vi "PathCreate.vi"(7 "Location":enum16{"CUMC", "SERI", "VMR", "Aline", "HSS"}(ring)=enum."Aline", 9 "Probe Name":string, 10 "Patient Info":T1 {"Plane" min=1 max=12 step=1 scale=0.0..12.0}, 11 "base path":path) -> (1 "FileName":string, 3 "appended path":path)   [LabVIEW 2022 SP3]
uses:
  PatientInfoDef.ctl
panel:
  in  "Frequency":i16
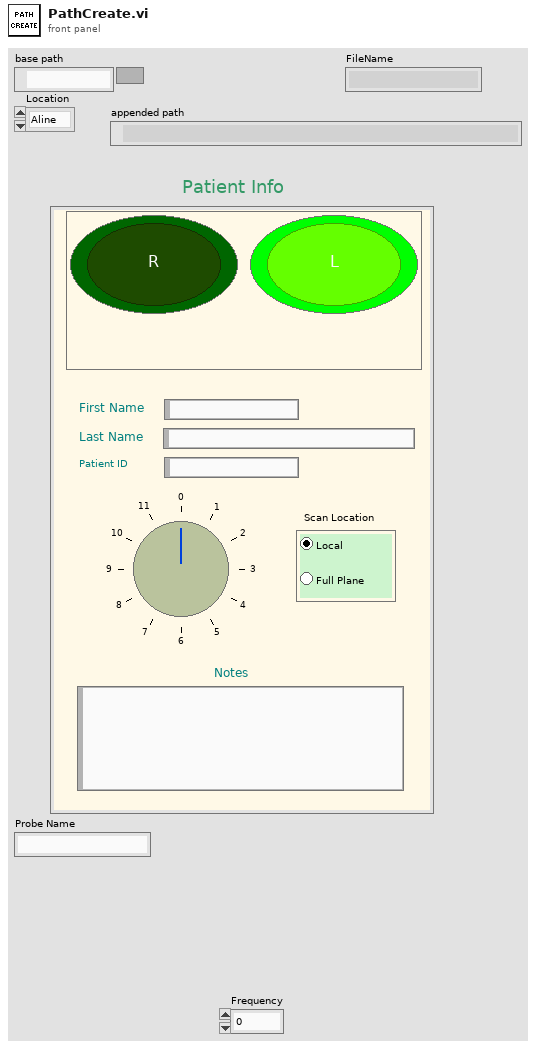
[diagram p1: front panel]
types:
  T1 = typedef "PatientInfoDef.ctl" = cluster{"Eye Selector":enum32{"Left", "Right"}, "Plane":i8, "First Name":string, "Last Name":string, "Notes":string, "Patient ID":string, "Scan Location":enum32{"Radio Selection 1", "Radio Selection 2"}}
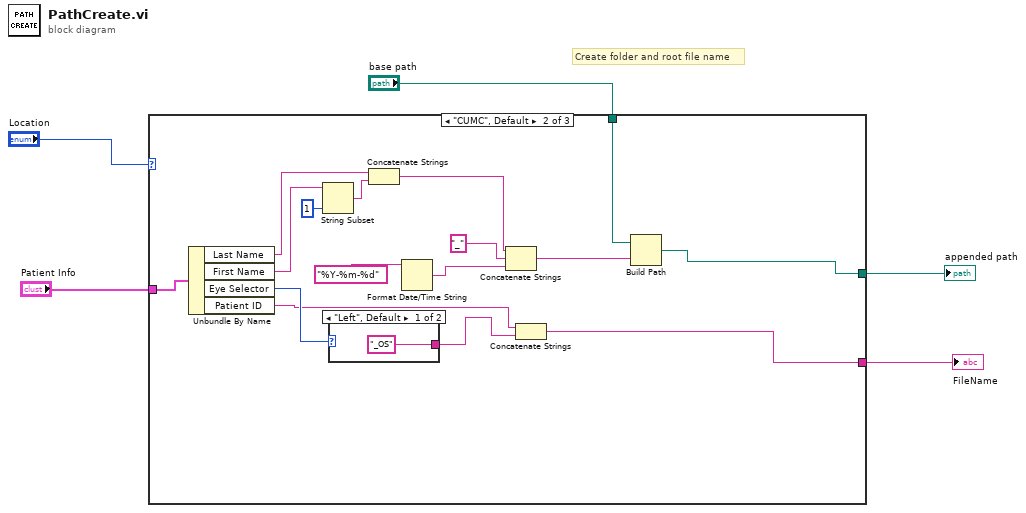
[diagram p0: block diagram]
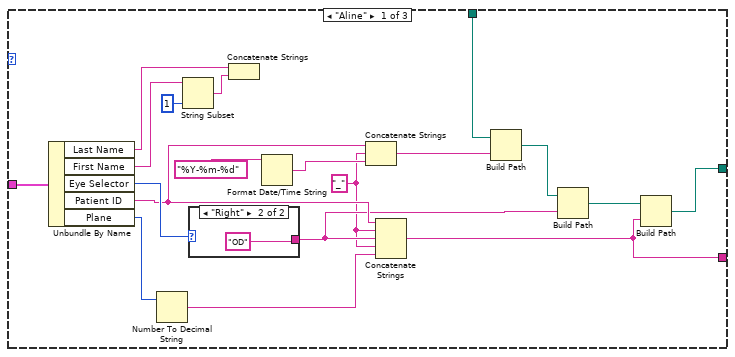
[diagram p2: hidden frame]
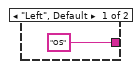
[diagram p3: hidden frame]
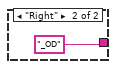
[diagram p4: hidden frame]
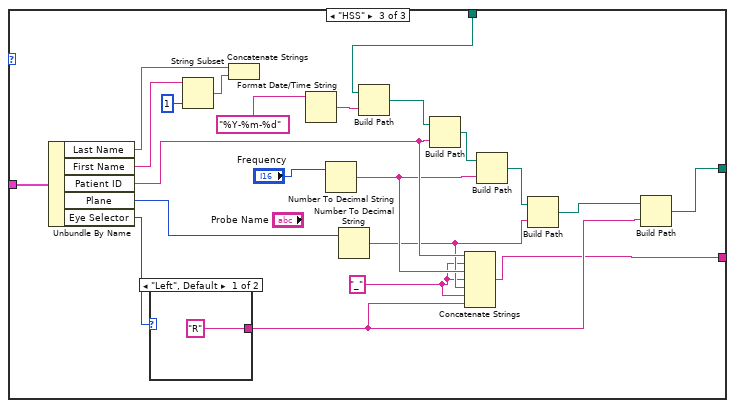
[diagram p5: hidden frame]
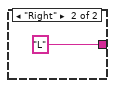
[diagram p6: hidden frame]
diagram:
  # "Create folder and root file name"
  n1 = case shown="\"CUMC\", Default" "Location" {
    tunnel: "base path" -> [w17 w35 w55]
    tunnel: "Patient Info" -> [w15 w33 w61]
    tunnel: [w7 w27 w58] -> w3
    tunnel: [w6 w30 w45] -> w2
    frame "Aline" {
      w9 = "_"
      n2 = Unbundle By Name(w15) -> ("Last Name"=w20:string, "First Name"=w22:string, "Eye Selector"=w23:enum32{"Left", "Right"}, "Patient ID"=w14:string, "Plane"=w11:i8)
      n3 = Number To Decimal String(number=w11) -> (decimal integer string=w10:string)  [unwired: 1 in]
      n4 = String Subset(string=w22, length (rest)=1 ("length (rest)")) -> (substring=w21:string)  [unwired: 1 in]
      n5 = case shown="\"Right\"" w23 {
        tunnel: ["OS" "OD"] -> w13
        frame "Left", Default {
        }
        frame "Right" {
        }
      }
      n6 = Concatenate Strings(w20, w21) -> ()  [unwired: 1 out]
      n7 = Format Date/Time String(time format string (%c)="%Y-%m-%d") -> (date/time string=w18:string)  [unwired: 2 in]
      n8 = Concatenate Strings(w14, w9, w18) -> (w16:string)
      n9 = Concatenate Strings(w14, w9, w13, w9, w10) -> (w6:string)
      n10 = Build Path(base path=w17, name or relative path=w16) -> (appended path=w12:path)
      n11 = Build Path(base path=w12, name or relative path=w13) -> (appended path=w8:path)
      n12 = Build Path(base path=w8, name or relative path=w6) -> (appended path=w7:path)
    }
    frame "CUMC", Default {
      n13 = Unbundle By Name(w33) -> ("Last Name"=w38:string, "First Name"=w40:string, "Eye Selector"=w41:enum32{"Left", "Right"}, "Patient ID"=w32:string)
      n14 = String Subset(string=w40, length (rest)=1 ("length (rest)")) -> (substring=w39:string)  [unwired: 1 in]
      n15 = case shown="\"Left\", Default" w41 {
        tunnel: ["_OS" "_OD"] -> w28
        frame "Left", Default {
        }
        frame "Right" {
        }
      }
      n16 = Concatenate Strings(w38, w39) -> (w29:string)
      n17 = Format Date/Time String(time format string (%c)="%Y-%m-%d") -> (date/time string=w36:string)  [unwired: 2 in]
      n18 = Concatenate Strings(w29, "_", w36) -> (w34:string)
      n19 = Concatenate Strings(w32, w28) -> (w30:string)
      n20 = Build Path(base path=w35, name or relative path=w34) -> (appended path=w27:path)
    }
    frame "HSS" {
      w47 = "_"
      n21 = Unbundle By Name(w61) -> ("Last Name"=w63:string, "First Name"=w65:string, "Patient ID"=w50:string, "Plane"=w59:i8, "Eye Selector"=w57:enum32{"Left", "Right"})
      n22 = case shown="\"Left\", Default" w57 {
        tunnel: ["R" "L"] -> w46
        frame "Left", Default {
        }
        frame "Right" {
        }
      }
      n23 = String Subset(string=w65, length (rest)=1 ("length (rest)")) -> (substring=w64:string)  [unwired: 1 in]
      n24 = Concatenate Strings(w63, w64) -> ()  [unwired: 1 out]
      n25 = Format Date/Time String(time format string (%c)="%Y-%m-%d") -> (date/time string=w56:string)  [unwired: 2 in]
      n26 = Number To Decimal String(number="Frequency") -> (decimal integer string=w49:string)  [unwired: 1 in]
      n27 = Number To Decimal String(number=w59) -> (decimal integer string=w48:string)  [unwired: 1 in]
      n28 = Build Path(base path=w55, name or relative path=w56) -> (appended path=w54:path)
      n29 = Build Path(base path=w54, name or relative path=w50) -> (appended path=w60:path)
      n30 = Concatenate Strings(w50, w47, w49, w47, w48, w47, w46) -> (w45:string)
      n31 = Build Path(base path=w60, name or relative path=w49) -> (appended path=w52:path)
      n32 = Build Path(base path=w52, name or relative path=w48) -> (appended path=w51:path)
      n33 = Build Path(base path=w51, name or relative path=w46) -> (appended path=w58:path)
    }
  }
  "appended path" <- w3
  "FileName" <- w2
